vi "生成CT表头.vi"() -> (3 "CT信息":T1)   [LabVIEW 2017]
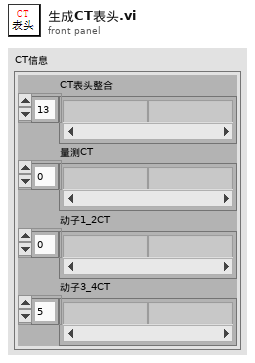
[diagram p1: front panel]
types:
  T1 = typedef "CT信息.ctl" = cluster{"CT表头整合":string[], "量测CT":string[], "动子1_2CT":string[], "动子3_4CT":string[]}
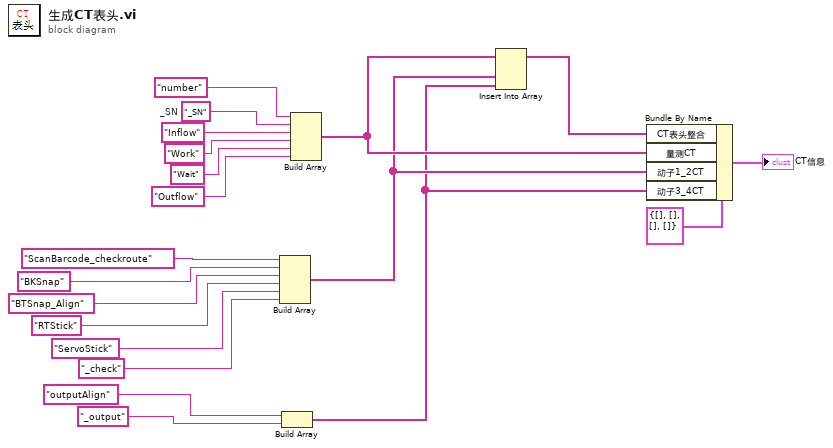
[diagram p0: block diagram]
diagram:
  w6 = "_SN"  # _SN
  n1 = Build Array("ScanBarcode_checkroute", "BKSnap", "BTSnap_Align", "RTStick", "ServoStick", "_check") -> (w8:string[])
  n2 = Build Array("outputAlign", "_output") -> (w1:string[])
  n3 = Build Array("number", w6, "Inflow", "Work", "Wait", "Outflow") -> (w9:string[])
  n4 = Insert Into Array(array=w9, new element #1=w8, new element #2=w1) -> (w7:string[])  [unwired: 1 in]
  n5 = Bundle By Name(cluster=T1 {"CT表头整合"=[], "量测CT"=[], "动子1_2CT"=[], "动子3_4CT"=[]} ("CT信息"), "CT表头整合"=w7, "量测CT"=w9, "动子1_2CT"=w8, "动子3_4CT"=w1) -> (→"CT信息":T1)
